vi "Protection and Counter Host Automation Example.vi"() -> ()   [LabVIEW 2019]
uses:
  <vilib>/xnet/xnet.llb/XNET Frame CAN.ctl
  <vilib>/xnet/xnet.llb/XNET Frame Type CAN.ctl
  Protection and Counter Host Automation API.lvlib
panel:
  out "error out":errorcluster
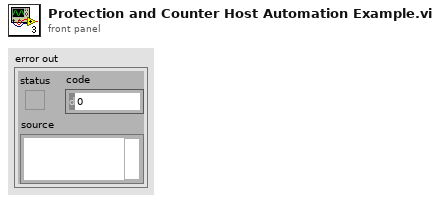
[diagram p1: front panel]
types:
  T1 = typedef "XNET Frame CAN.ctl" = cluster{"timestamp":timestamp, "payload":u8[], "identifier":u32, "type":T2, "extended?":bool, "echo?":bool}
  T2 = typedef "XNET Frame Type CAN.ctl" = u8
  T3 = typedef "Protection and Counter Host Automation API.lvlib/API Variables.ctl" = cluster{"TCP Comm":T4}
  T4 = typedef "NI STM.lvlib/TCP Connection Info.ctl" = cluster{"connection ID":refnum<k5>, "meta data":T5[]}
  T5 = typedef "NI STM.lvlib/MetaDataElement.ctl" = string
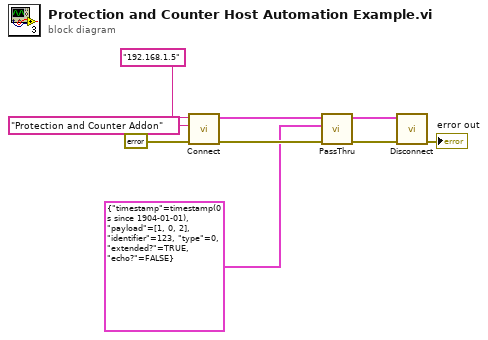
[diagram p0: block diagram]
diagram:
  n1 = call "Connect.vi"("error in (no error)"=errorcluster {"status"=FALSE, "code"=0, "source"=""}, "Addon Name"="Protection and Counter Addon", "Address"="192.168.1.5") -> ("error out"=w6:errorcluster, "Ref"=w9:T3)  [unwired: 7 in]
  n2 = call "PassThru.vi"("error in (no error)"=w6, "Frame"=T1 {"timestamp"=timestamp(0 s since 1904-01-01), "payload"=[1, 0, 2], "identifier"=123, "type"=0, "extended?"=TRUE, "echo?"=FALSE}, "Ref in"=w9) -> ("error out"=w7:errorcluster, "Ref out"=w8:T3)  [unwired: 7 in]
  n3 = call "Disconnect.vi"("error in (no error)"=w7, "Ref"=w8) -> ("error out"=→"error out":errorcluster)  [unwired: 9 in]
